vi "From Variant.vi"(8 "Error In":errorcluster, 10 "Variant":variant, 11 "TD Flt In":refnum<class "Flt.lvclass">) -> (0 "Error Out":errorcluster, 3 "TD Flt Out":refnum<class "Flt.lvclass">)   [LabVIEW 2017, in "Tree API.lvlib" / "Flt.lvclass"]
doc: "Dynamic dispatch interface for conversion of variant LV data to Tree Data classes."
uses:
  Flt.lvclass
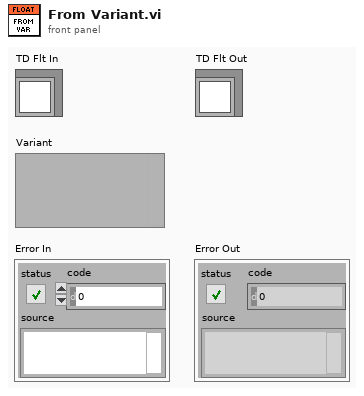
[diagram p1: front panel]
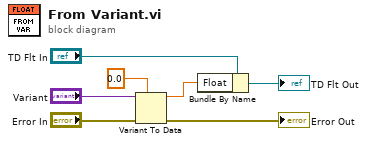
[diagram p0: block diagram]
diagram:
  n1 = Variant To Data(error in="Error In", type=0.0 ("Float"), Variant="Variant") -> (data=w1:dbl, error out=→"Error Out":errorcluster)
  n2 = Bundle By Name(cluster="TD Flt In", "Float"=w1) -> (→"TD Flt Out":refnum<class "Flt.lvclass">)
